vi "GV-DrawYaxis.vi"(6 "Picture IN":picture, 8 "error in (no error)":errorcluster, 9 "X-position":i16, 10 "Plot":i32, 11 "Gviewer in":refnum<class "Gviewer.lvclass">) -> (0 "error out":errorcluster, 3 "Gviewer out":refnum<class "Gviewer.lvclass">, 4 "Picture OUT":picture)   [LabVIEW 2020, in "Sgraph_lib_V1.lvlib" / "Gviewer.lvclass"]
doc: "Draw an Y-scale on the graph canvas"
uses:
  Gviewer.lvclass
  Gviewer.lvclass/Gviewer.ctl
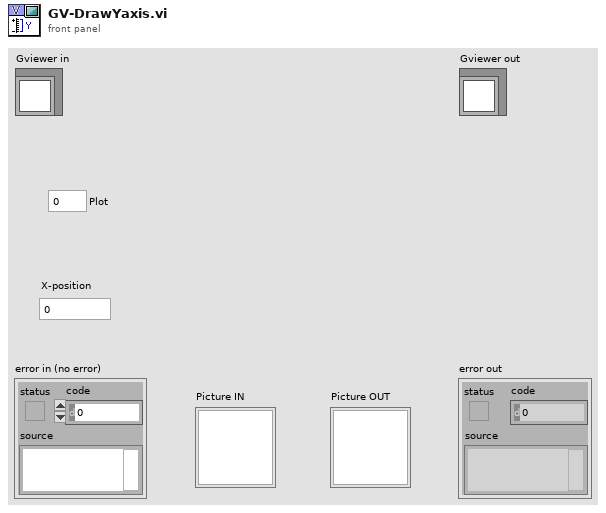
[diagram p1: front panel]
types:
  T1 = cluster{"coordinate 1":i16, "value 1":dbl, "coordinate 2":i16, "value 2":dbl, "log?(F)":bool}
  T2 = cluster{"horizontal":bool, "left/top":bool, "draw bar":bool, "line color":u32, "text color(black)":u32}
  T3 = cluster{"data":dbl[], "max":dbl[], "min":dbl[], "Status":u32[]}[]
  T4 = typedef "Sgraph_lib_V1.lvlib/Gviewer.lvclass/Typedef_SelProperties.ctl" = cluster{"Color":u32, "LineType":T5, "max":dbl, "min":dbl, "unit":string}
  T5 = typedef "Sgraph_lib_V1.lvlib/Gviewer.lvclass/Typedef_LineType.ctl" = enum16{"num_bare", "num_MinMax_Area", "num_MinMax_Lines", "num_MinMax_Forfor", "num_Max_Area", "num_Max_Line", "num_Max_Forfor", "num_Min_Area", "num_Min_Line", "num_Min_Fosfor", "Boolean_Line_01", "Boolean_Area_01", "Boolean_Fosfor_01", "Boolean_Line_TF", "Boolean_Area_TF", "Boolean_Fosfor_TF", "Boolean_OnOff_Line", "Boolean_OnOff_Area", "Boolean_OnOff_Fosfor", "Boolean_spare", "StringEvent_Line", "StringEvent_TimeLine"}
  T6 = cluster{"data":dbl[], "max":dbl[], "min":dbl[], "Status":u32[]}
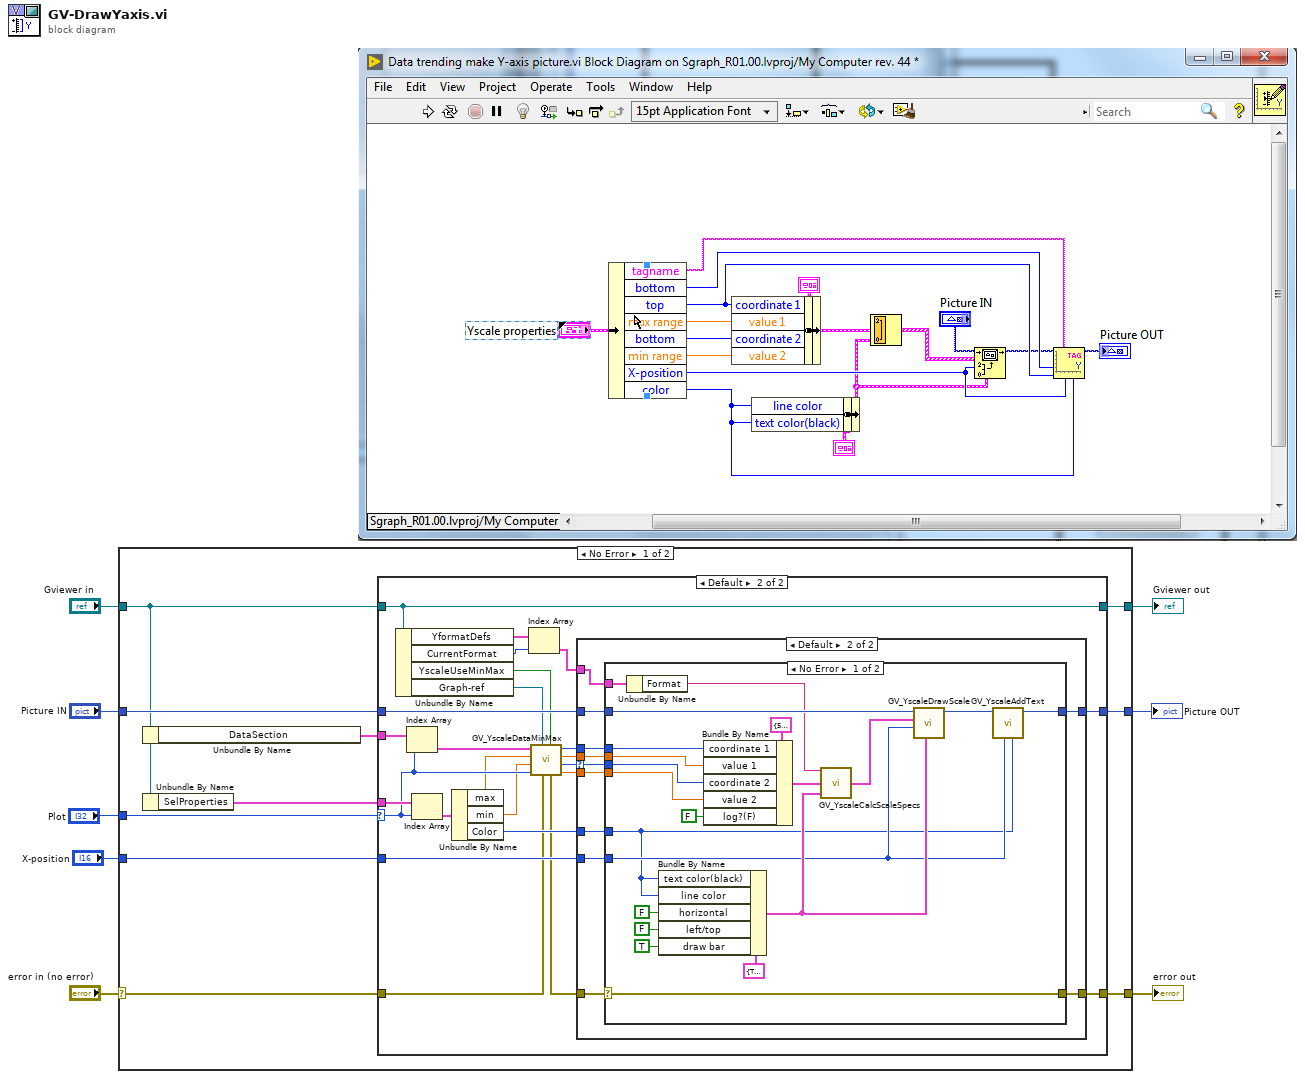
[diagram p0: block diagram]
diagram:
  n1 = case shown="No Error" "error in (no error)" {
    selector: "error in (no error)" -> [w11 w84]
    tunnel: [w10 w84] -> w7
    tunnel: [w9 w83] -> w5
    tunnel: "Gviewer in" -> [w13 w83]
    tunnel: "Picture IN" -> [w17 w82]
    tunnel: [w18 w82] -> w3
    tunnel: "X-position" -> [w16 _]
    tunnel: "Plot" -> [w12 _]
    frame No Error {
      n2 = Unbundle By Name(w13) -> ("DataSection"=w14:T3)
      n3 = Unbundle By Name(w13) -> ("SelProperties"=w15:T4[])
      n4 = case shown="Default" w12 {
        selector: w12 -> [_ w35]
        tunnel: [w20 w45] -> w18
        tunnel: w17 -> [w20 w44]
        tunnel: w16 -> [_ w43]
        tunnel: w15 -> [_ w42]
        tunnel: w14 -> [_ w39]
        tunnel: w13 -> [w21 w31]
        tunnel: w11 -> [w19 w34]
        tunnel: [w19 w29] -> w10
        tunnel: [w21 w31] -> w9
        frame -1 {
        }
        frame Default {
          n5 = Unbundle By Name(w31) -> ("YformatDefs"=w26:cluster{"Description":string, "Format":string}[], "CurrentFormat"=w25:i32, "YscaleUseMinMax"=w22:bool, "Graph-ref"=w23:refnum<vi>)
          n6 = Index Array(array=w39, index=w35) -> (element=w38:T6)
          n7 = Index Array(array=w42, index=w35) -> (element=w41:T4)
          n8 = Unbundle By Name(w41) -> ("max"=w28:dbl, "min"=w27:dbl, "Color"=w40:u32)
          n9 = Index Array(array=w26, index=w25) -> (element=w24:cluster{"Description":string, "Format":string})
          n10 = call "GV_YscaleDataMinMax.vi"("IncludeMinMax"=w22, "error in (no error)"=w34, "Graph-ref"=w23, "Plot"=w35, "Scale-min"=w27, "Scale-max"=w28, "PAQ-data"=w38) -> ("min"=w36:dbl, "Coord-min"=w32:i32, "max"=w37:dbl, "Coord-max"=w33:i32, "error out"=w30:errorcluster)
          n11 = case shown="Default" w32 {
            selector: w32 -> [_ w51]
            tunnel: [w47 w58] -> w45
            tunnel: w44 -> [w47 w57]
            tunnel: w43 -> [_ w56]
            tunnel: w40 -> [_ w55]
            tunnel: w37 -> [_ w54]
            tunnel: w36 -> [_ w53]
            tunnel: w33 -> [_ w52]
            tunnel: w30 -> [w46 w50]
            tunnel: [w46 w49] -> w29
            tunnel: w24 -> [_ w48]
            frame -1 {
            }
            frame Default {
              n12 = case shown="No Error" w50 {
                selector: w50 -> [w61 w81]
                tunnel: [w77 w80] -> w58
                tunnel: w57 -> [w76 w80]
                tunnel: w56 -> [w73 _]
                tunnel: w55 -> [w69 _]
                tunnel: w54 -> [w65 _]
                tunnel: w53 -> [w64 _]
                tunnel: w52 -> [w63 _]
                tunnel: w51 -> [w62 _]
                tunnel: [w61 w81] -> w49
                tunnel: w48 -> [w60 _]
                frame No Error {
                  n13 = Unbundle By Name(w60) -> ("Format"=w59:string)
                  n14 = Bundle By Name(cluster=T2 {"horizontal"=TRUE, "left/top"=FALSE, "draw bar"=FALSE, "line color"=0, "text color(black)"=0} ("scale attributes"), "text color(black)"=w69, "line color"=w69, "horizontal"=FALSE, "left/top"=FALSE, "draw bar"=TRUE) -> (w74:T2)
                  n15 = Bundle By Name(cluster=T1 {"coordinate 1"=5, "value 1"=5.0, "coordinate 2"=5, "value 2"=5.0, "log?(F)"=FALSE} ("scale definition"), "coordinate 1"=w63, "value 1"=w65, "coordinate 2"=w62, "value 2"=w64, "log?(F)"=FALSE) -> (w67:T1)
                  n16 = call "GV_YscaleCalcScaleSpecs.vi"("FormatString"=w59, "scale definition"=w67, "scale attributes"=w74) -> ("scale specs"=w79:cluster{"coordinate":i16, "label":string}[])  [unwired: 6 in]
                  n17 = call "GV_YscaleDrawScale.vi"("scale attributes"=w74, "constant coordinate"=w73, "scale specs"=w79, "picture"=w76) -> ("new picture"=w78:picture)  [unwired: 7 in]
                  n18 = call "GV_YscaleAddText.vi"("Color"=w69, "X-position"=w73, "2D Picture IN"=w78) -> ("2D Picture OUT"=w77:picture)  [unwired: 8 in]
                }
                frame Error {
                }
              }
            }
          }
        }
      }
    }
    frame Error {
    }
  }
  "error out" <- w7
  "Gviewer out" <- w5
  "Picture OUT" <- w3
